vi "Edge with init.vi"(7 "init":bool, 11 "in":bool) -> (3 "out":bool)   [LabVIEW 2019, in "Stand.lvclass"]
uses:
  Stand.lvclass
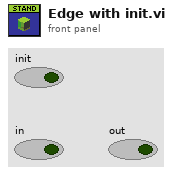
[diagram p1: front panel]
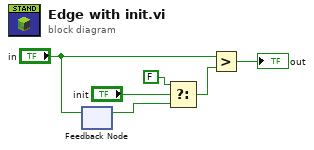
[diagram p0: block diagram]
diagram:
  n1 = feedback-in #1("in") -> ()
  n2 = feedback #1() -> (w3:bool)  [unwired: 1 in]
  n3 = Select(t=FALSE, s="init", f=w3) -> (s? t:f=w1:bool)
  n4 = Greater?(x="in", y=w1) -> (0:→"out":bool)
